vi "getSignalsRecursive.vi"(8 "error in (no error)":errorcluster, 11 "IDevice in":refnum<class "IDevice.lvclass">) -> (0 "error out":errorcluster, 2 "Available Sigals out":refnum<class "ISignal.lvclass">[](array[class]), 3 "IDevice out":refnum<class "IDevice.lvclass">)   [LabVIEW 2022 SP3, in "openDAQ.lvlib" / "IBaseObject.lvlib" / "IPropertyObject.lvlib" / "IComponent.lvlib" / "IFolder.lvlib" / "IDevice.lvlib" / "IDevice.lvclass"]
uses:
  <instrlib>/openDAQ/Public/Classes/IDevice/IDevice.lvclass
  <instrlib>/openDAQ/Public/Classes/IDevice/IDevice.lvclass/IDevice.ctl
  <instrlib>/openDAQ/Public/Classes/daqCoreTypes/IList/IList.lvclass
  <instrlib>/openDAQ/Public/Classes/daqCoreTypes/IList/Polymorphic/getList/getSignalList.vi
  <instrlib>/openDAQ/Binaries/Windows/x86/copendaq32.dll
  <instrlib>/openDAQ/Public/Classes/ISignal/ISignal.lvclass
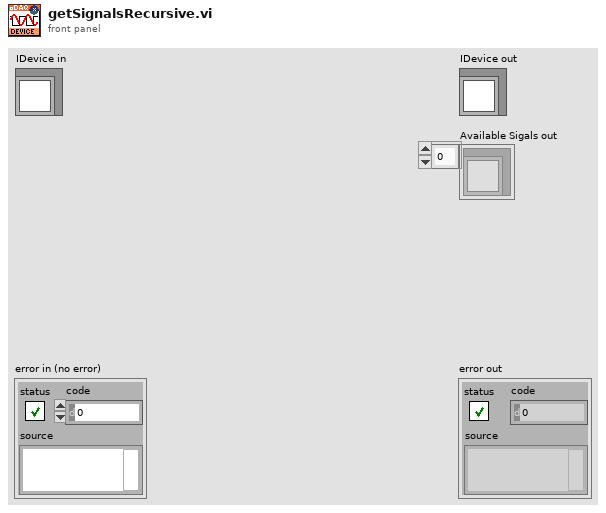
[diagram p1: front panel]
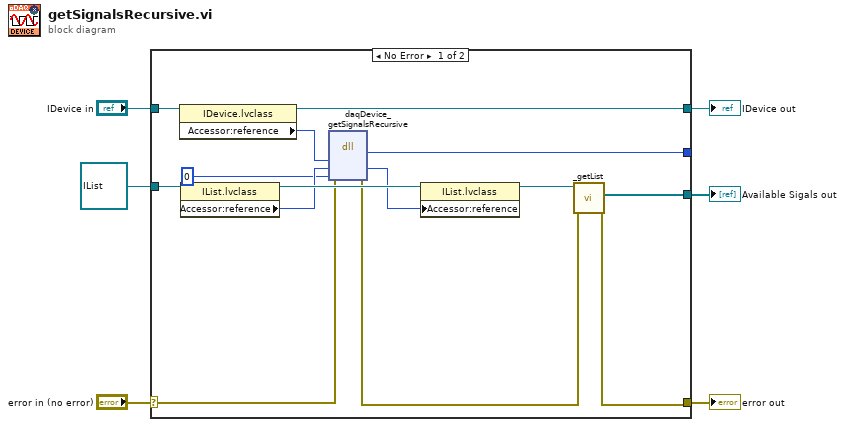
[diagram p0: block diagram]
diagram:
  n1 = case shown="No Error" "error in (no error)" {
    selector: "error in (no error)" -> [w13 w22]
    tunnel: [w9 w22] -> w5
    tunnel: [w18 w21] -> w3
    tunnel: "IDevice in" -> [w19 w21]
    tunnel: refnum<class "IList.lvclass"> refnum ("openDAQ.lvlib:daqCoreTypes.lvlib:IList.lvclass") -> [w16 _]
    tunnel: [w11 _] -> w1
    tunnel: [w7 _] -> _
    frame No Error {
      n2 = property class="IDevice.lvclass"(reference=w19) -> (reference out=w18:refnum<class "IDevice.lvclass">, "Accessor:reference"=w17:i64)  [unwired: 1 in, 1 out]
      n3 = property class="IList.lvclass"(reference=w16) -> (reference out=w20:refnum<class "IList.lvclass">, "Accessor:reference"=w15:i64)  [unwired: 1 in, 1 out]
      n4 = dll-call lib="C:/Program Files (x86)/National Instruments/LabVIEW 2022/instr.lib/openDAQ/Binaries/Windows/x86/copendaq*.*" fn="daqDevice_getSignalsRecursive"(error in=w13, "device"=w17, "signals"=w15, "searchFilter"=i64 0) -> (error out=w10:errorcluster, "return type"=w7:u32, "signals"=w14:i64)  [unwired: 4 in, 1 out]
      n5 = property class="IList.lvclass"(reference=w20, "Accessor:reference"=w14) -> (reference out=w12:refnum<class "IList.lvclass">)  [unwired: 1 in, 1 out]
      n6 = call-poly <instrlib>:"_getList.vi"("error in (no error)"=w10, "IList in"=w12) -> ("error out"=w9:errorcluster, "devices out"=w11:refnum<class "ISignal.lvclass">[])  [unwired: 8 in]
    }
    frame Error {
    }
  }
  "error out" <- w5
  "IDevice out" <- w3
  "Available Sigals out" <- w1
